vi "Waveforms to 2D DBL Array.vi"(11 "wavefrms":waveform(dbl)[](array[waveform])) -> (3 "2D DBL array":dbl[][](array[numeric]))   [LabVIEW 2013, in "varilib.lvlib"]
doc: "Converts waveform array to array of doubles with following format:\n(T1 X1 Y1 Z1 ... )\n(T2 X2 Y2 Z2 ... )\n...\n(Tend Xend Yend Zend ... )\nwhere T series is relative starting with 0 time. VI suppose all waveforms has the same length and are sampled at the same time."
uses:
  varilib.lvlib
  <vilib>/Waveform/WDTOps.llb/WDT Get Waveform Time Array DBL.vi
panel:
  out "t0":timestamp
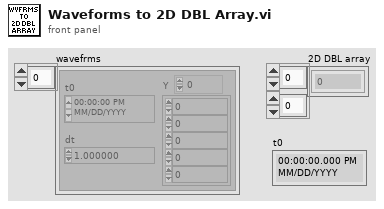
[diagram p1: front panel]
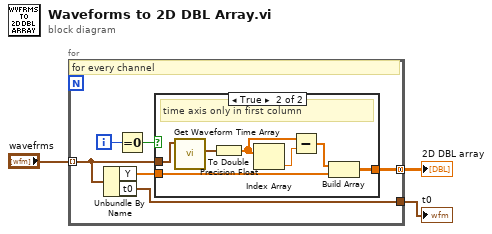
[diagram p0: block diagram]
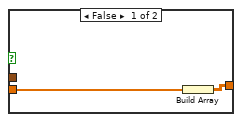
[diagram p2: hidden frame]
diagram:
  n1 = for {
    tunnel: [w5] -> w3 mode=concatenating
    tunnel: "wavefrms" -> [w9] mode=indexing
    tunnel: [w4] -> w1
    i -> [w8]
    # "for every channel"
    n2 = Unbundle By Name(w9) -> ("Y"=w6:dbl[], "t0"=w4:timestamp)
    n3 = Equal To 0?(x=w8) -> (x = 0?=w7:bool)
    n4 = case shown="True" w7 {
      tunnel: w9 -> [_ w18]
      tunnel: w6 -> [w11 w13]
      tunnel: [w10 w12] -> w5
      frame False {
        n5 = Build Array(w11) -> (w10:dbl[][])
      }
      frame True {
        # "time axis only in first column"
        n6 = call-poly <vilib>:"Get Waveform Time Array.vi"("waveform in"=w18) -> ("X array"=w15:timestamp[])  [unwired: 9 in, 1 out]
        n7 = To Double Precision Float(number=w15) -> (double precision float=w16:dbl[])
        n8 = Index Array(array=w16) -> (element=w17:dbl)  [unwired: 1 in]
        n9 = Subtract(x=w16, y=w17) -> (x-y=w14:dbl[])
        n10 = Build Array(w14, w13) -> (w12:dbl[][])
      }
    }
  }
  "2D DBL array" <- w3
  "t0" <- w1
